vi "DoubleClickCallback.vi"(4 "NotifyIcon in":refnum<class "MGI_TrayIcon.lvclass">, 5 "Event Data":cluster{"sender":refnum<k24>, "e":refnum<k24>}, 6 "Control Ref":refnum<k24>, 7 "Event Common Data":T1) -> ()   [LabVIEW 2016, in "MGI_TrayIcon.lvclass"]
doc: "Called when the tray icon is double clicked. This will look at the menu structure for an Item with DefaultItem set to true. If an item is found, it will perform a click action on it.\n\nAuthored by Derek E. Trepanier\nsupport@mooregoodideas.com\nwww.mooregoodideas.com\n\nCopyright (c) 2012, Moore Good Ideas, Inc.\n\nAll rights reserved.\n\nRedistribution and use in source and binary forms, with or without modification, are permitted provided that the following conditions are met:\n\n * Redistributions of source code must retain the above copyright notice, this list of conditions and the following disclaimer.\n * Redistributions in binary form must reproduce the above copyright notice, this list of conditions and the following disclaimer in the documentation and/or other materials provided with the distribution.\n * Neither the name of Moore Good Ideas, Inc. nor the names of its contributors may be used to endorse or promote products derived from this software without specific prior written permission.\n\nTHIS SOFTWARE IS PROVIDED BY THE COPYRIGHT HOLDERS AND CONTRIBUTORS \"AS IS\" AND ANY EXPRESS OR IMPLIED WARRANTIES, INCLUDING, BUT NOT LIMITED TO, THE IMPLIED WARRANTIES OF MERCHANTABILITY AND FITNESS FOR A PARTICULAR PURPOSE ARE DISCLAIMED. IN NO EVENT SHALL THE COPYRIGHT OWNER OR CONTRIBUTORS BE LIABLE FOR ANY DIRECT, INDIRECT, INCIDENTAL, SPECIAL, EXEMPLARY, OR CONSEQUENTIAL DAMAGES (INCLUDING, BUT NOT LIMITED TO, PROCUREMENT OF SUBSTITUTE GOODS OR SERVICES; LOSS OF USE, DATA, OR PROFITS; OR BUSINESS INTERRUPTION) HOWEVER CAUSED AND ON ANY THEORY OF LIABILITY, WHETHER IN CONTRACT, STRICT LIABILITY, OR TORT (INCLUDING NEGLIGENCE OR OTHERWISE) ARISING IN ANY WAY OUT OF THE USE OF THIS SOFTWARE, EVEN IF ADVISED OF THE POSSIBILITY OF SUCH DAMAGE."
uses:
  <userlib>/_MGI/Menu Building/MenuTypes/TrayIcon/MGI_TrayIcon.lvclass
  System.Windows.Forms
  C:/Program Files (x86)/National Instruments/LabVIEW 2016/user.lib/_MGI/Menu Building/MenuTypes/MGI_Menu.lvclass
  <userlib>/_MGI/Menu Building/MenuItem/TrayIcon/MGI_TrayItem.lvclass
  C:/Program Files (x86)/National Instruments/LabVIEW 2016/user.lib/_MGI/Menu Building/MenuItem/MGI_MenuItem.lvclass
  <userlib>/_MGI/Menu Building/MenuTypes/Read Menu Items.vi
  <userlib>/_MGI/Menu Building/MenuItem/TrayIcon/Read DefaultItem.vi
  <userlib>/_MGI/Menu Building/MenuItem/MGI_MenuItem.lvclass
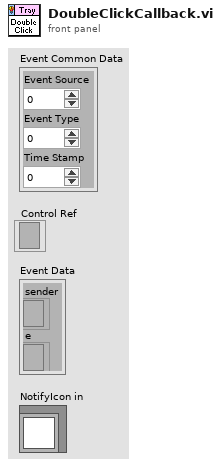
[diagram p1: front panel]
types:
  T1 = cluster{"Event Source":i32, "Event Type":u32, "Time Stamp":u32}
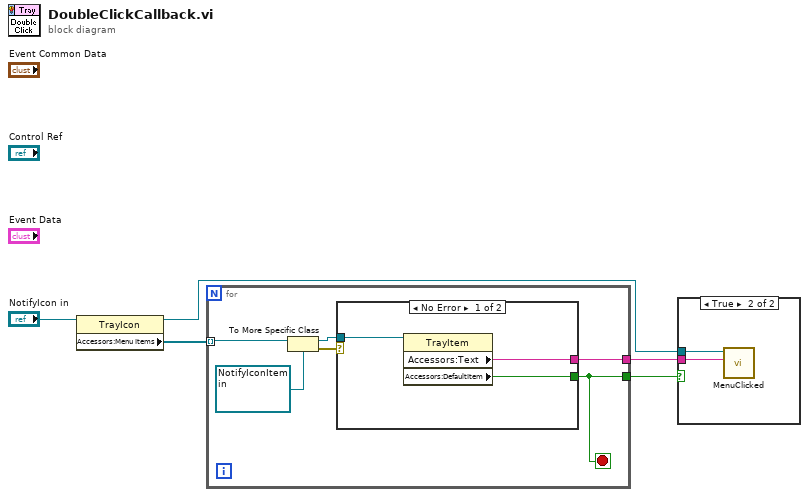
[diagram p0: block diagram]
diagram:
  n1 = property class="TrayIcon"(reference="NotifyIcon in") -> (reference out=w2:refnum<class "MGI_TrayIcon.lvclass">, "Accessors:Menu Items"=w4:refnum<data-value>[])  [unwired: 1 in, 1 out]
  n2 = for {
    tunnel: w4 -> [w11] mode=indexing
    tunnel: [w8] -> w3
    tunnel: [w7] -> w1
    stop <- w7 stop-if-true
    n3 = To More Specific Class(target class=refnum<data-value> refnum ("Notify Icon Item"), reference=w11) -> (specific class reference=w9:refnum<data-value>, error out=w10:errorcluster)  [unwired: 1 in]
    n4 = case shown="No Error" w10 {
      tunnel: w9 -> [w14 _]
      tunnel: [w13 _] -> w7
      tunnel: [w12 _] -> w8
      frame No Error {
        n5 = property class="TrayItem"(reference=w14) -> ("Accessors:Text"=w12:string, "Accessors:DefaultItem"=w13:bool)  [unwired: 1 in, 2 out]
      }
      frame Error {
      }
    }
  }
  n6 = case shown="True" w1 {
    tunnel: w3 -> [_ w16]
    tunnel: w2 -> [_ w15]
    frame False {
    }
    frame True {
      n7 = call-dynamic "MenuClicked.vi"("Full Tag"=w16, "Menu in"=w15) -> ()  [unwired: 8 in, 2 out]
    }
  }
